vi "Get First Row with Smaller Index.vi"(8 "error in":errorcluster, 10 "Row Index":u32, 11 "SheetData in":refnum<k24>) -> (0 "error out":errorcluster, 1 "Smaller Row Index":u32, 2 "Row":refnum<k24>, 3 "SheetData out":refnum<k24>)   [LabVIEW 2019, in "Open Xml.lvlib"]
uses:
  Open Xml.lvlib
  D:/git/Open-Xml-LabVIEW/Source/DocumentFormat.OpenXml.dll
  DocumentFormat.OpenXml.dll
  D:/git/Open-Xml-LabVIEW/Source/DocumentFormat.OpenXml.Framework.dll
  DocumentFormat.OpenXml.Framework.dll
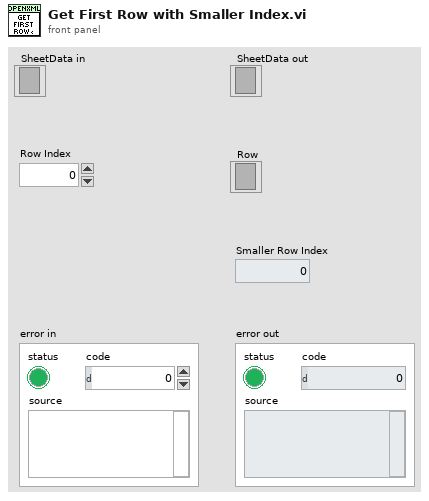
[diagram p1: front panel]
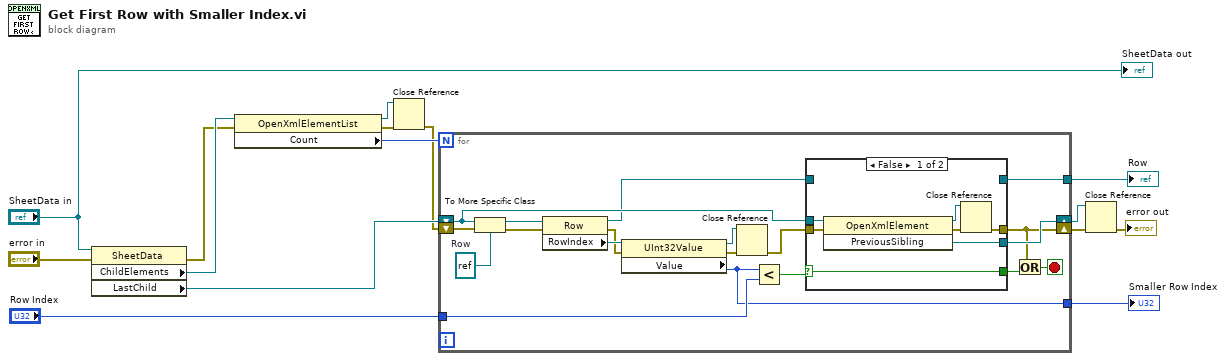
[diagram p0: block diagram]
diagram:
  n1 = property class="SheetData"(reference="SheetData in", error in="error in") -> (error out=w3:errorcluster, "ChildElements"=w9:refnum<k24>, "LastChild"=w7:refnum<k24>)  [unwired: 1 out]
  n2 = property class="OpenXmlElementList"(reference=w9, error in=w3) -> (reference out=w6:refnum<k24>, error out=w5:errorcluster, "Count"=w8:i32)
  n3 = Close Reference(reference=w6, error in (no error)=w5) -> (error out=w4:errorcluster)
  n4 = for {
    N: w8 -> [_]
    shift-right: [w26] -> w1
    shift-left: w7 -> [w27]
    tunnel: "Row Index" -> [w30]
    tunnel: [w22] -> w13
    shift-right: [w25] -> w2
    shift-left: w4 -> [w33]
    tunnel: [w20] -> w10
    stop <- w29 stop-if-true
    w34 = refnum<k24> refnum  # Row
    n5 = To More Specific Class(target class=w34, reference=w27, error in=w33) -> (specific class reference=w31:refnum<k24>, error out=w32:errorcluster)
    n6 = property class="Row"(reference=w31, error in=w32) -> (reference out=w23:refnum<k24>, error out=w18:errorcluster, "RowIndex"=w19:refnum<k24>)
    n7 = property class="UInt32Value"(reference=w19, error in=w18) -> (reference out=w16:refnum<k24>, error out=w17:errorcluster, "Value"=w20:u32)
    n8 = Close Reference(reference=w16, error in (no error)=w17) -> (error out=w28:errorcluster)
    n9 = Less?(x=w20, y=w30) -> (x < y?=w21:bool)
    n10 = case shown="False" w21 {
      selector: w21 -> [w35 w43]
      tunnel: w28 -> [w41 w44]
      tunnel: w27 -> [w40 _]
      tunnel: [w38 _] -> w26
      tunnel: [w36 w44] -> w25
      tunnel: [w35 w43] -> w24
      tunnel: w23 -> [_ w42]
      tunnel: [_ w42] -> w22
      frame False {
        n11 = invoke class="OpenXmlElement" method="PreviousSibling"(reference=w40, error in=w41) -> (reference out=w39:refnum<k24>, error out=w37:errorcluster, "PreviousSibling"=w38:refnum<k24>)  [unwired: 1 in]
        n12 = Close Reference(reference=w39, error in (no error)=w37) -> (error out=w36:errorcluster)
      }
      frame True {
      }
    }
    n13 = Or(x=w25, y=w24) -> (x .or. y?=w29:bool)
  }
  "Row" <- w13
  "Smaller Row Index" <- w10
  n14 = Close Reference(reference=w1, error in (no error)=w2) -> (error out=→"error out":errorcluster)
  "SheetData out" <- "SheetData in"
